vi "数据写入位置.vi"(1 "标准值位置":string) -> (0 "显示值位置":string)   [LabVIEW 2015]
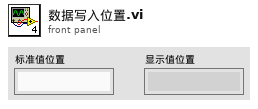
[diagram p1: front panel]
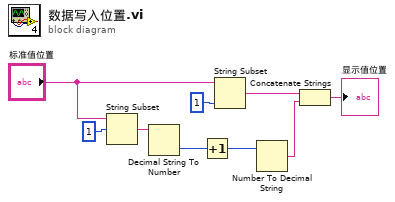
[diagram p0: block diagram]
diagram:
  n1 = String Subset(string="标准值位置", offset (0)=1 ("偏移量(0)")) -> (substring=w2:string)  [unwired: 1 in]
  n2 = Decimal String To Number(string=w2) -> (number=w3:i32)  [unwired: 2 in, 1 out]
  n3 = Increment(x=w3) -> (x+1=w5:i32)
  n4 = String Subset(string="标准值位置", length (rest)=1 ("长度（剩余）")) -> (substring=w7:string)  [unwired: 1 in]
  n5 = Number To Decimal String(number=w5) -> (decimal integer string=w6:string)  [unwired: 1 in]
  n6 = Concatenate Strings(w7, w6) -> (→"显示值位置":string)
